vi "Rysuj_obwiednie.vi"(8 "error in (no error)":errorcluster, 11 "Bufor in":T1) -> (0 "error out":errorcluster, 3 "Bufor out":T1)   [LabVIEW 2014]
doc: "Rysuje obwiednie dla przebiegów analogowych"
uses:
  Kontrolki/Przetwarzanie/Kanaly.ctl
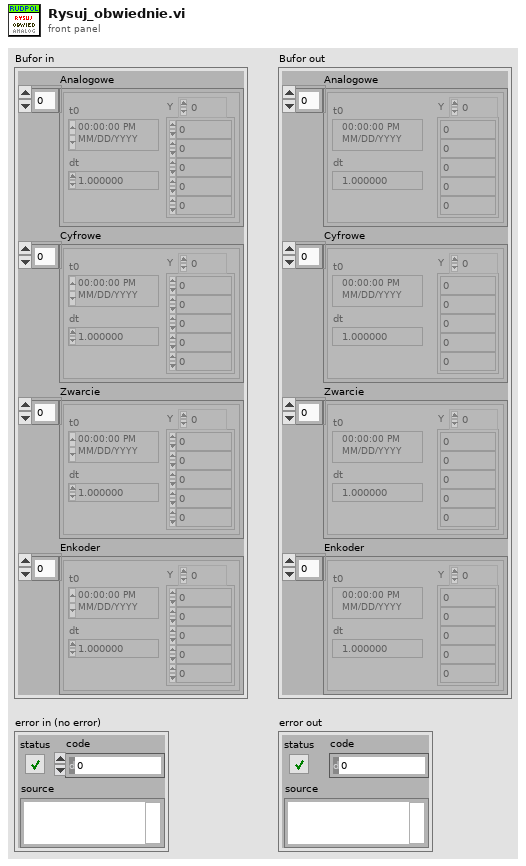
[diagram p1: front panel]
types:
  T1 = typedef "Kanaly.ctl" = cluster{"Analogowe":waveform(dbl)[], "Cyfrowe":waveform(dbl)[], "Zwarcie":waveform(dbl)[], "Enkoder":waveform(dbl)[]}
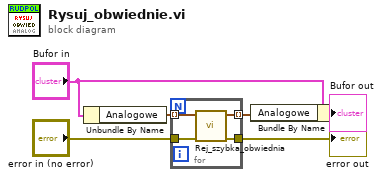
[diagram p0: block diagram]
diagram:
  n1 = Unbundle By Name("Bufor in") -> ("Analogowe"=w1:waveform(dbl)[])
  n2 = for {
    tunnel: w1 -> [w10] mode=indexing
    tunnel: [w9] -> w2 mode=indexing
    tunnel: [w8] -> w3
    tunnel: "error in (no error)" -> [w7]
    n3 = call "Rej_szybka_obwiednia.vi"("error in (no error)"=w7, "Wfm in"=w10) -> ("error out"=w8:errorcluster, "Wfm max out"=w9:waveform(dbl))  [unwired: 7 in, 1 out]
  }
  "error out" <- w3
  n4 = Bundle By Name(cluster="Bufor in", "Analogowe"=w2) -> (→"Bufor out":T1)
